vi "LS372_setup.vi"   [LabVIEW 2016]
uses:
  Instrument_Setup.vi
  Lake Shore 372/Lake Shore 372.lvlib
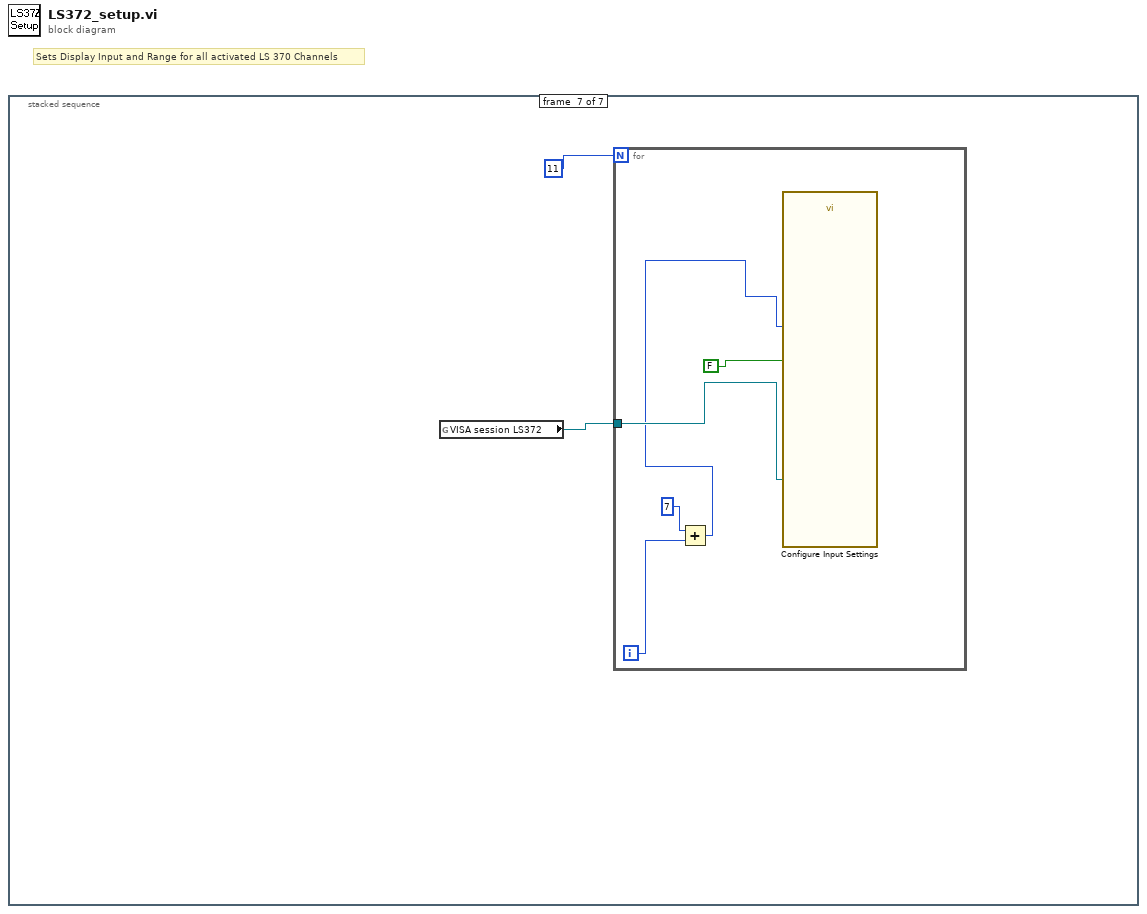
[diagram p0: block diagram]
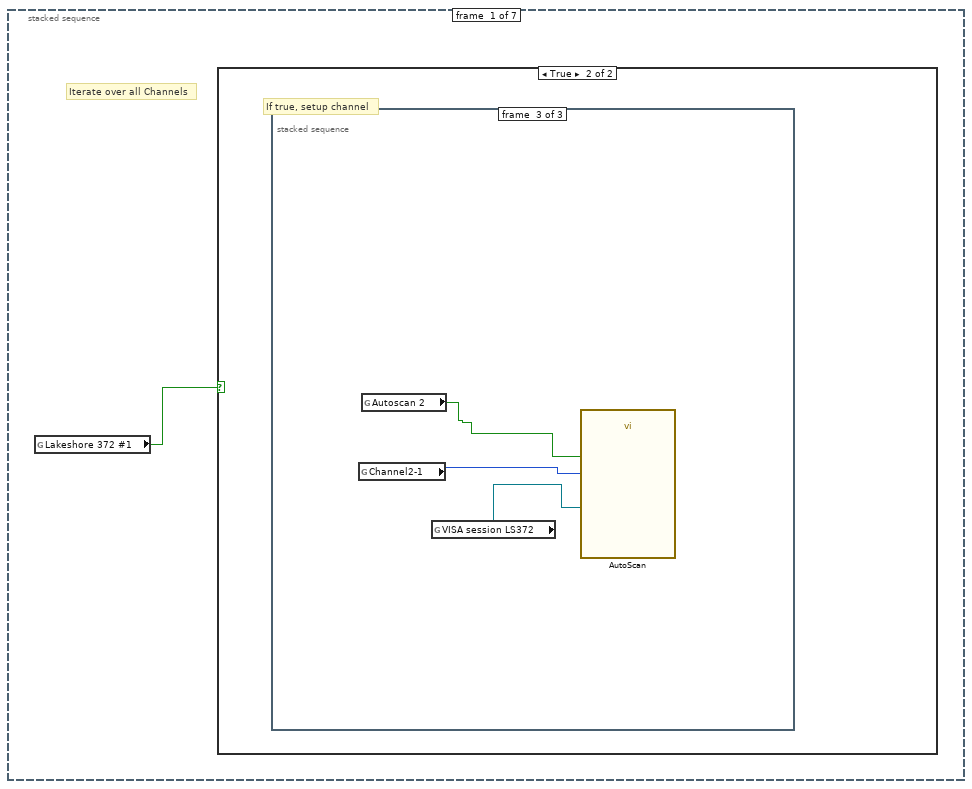
[diagram p2: hidden frame]
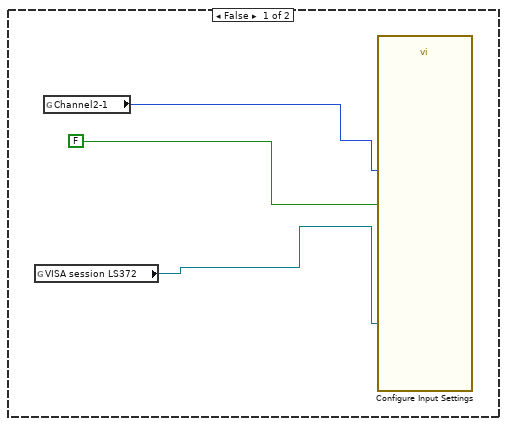
[diagram p3: hidden frame]
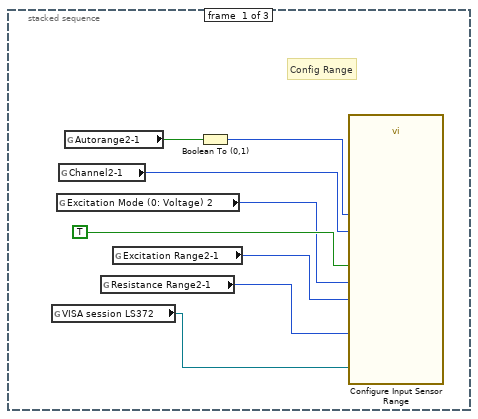
[diagram p4: hidden frame]
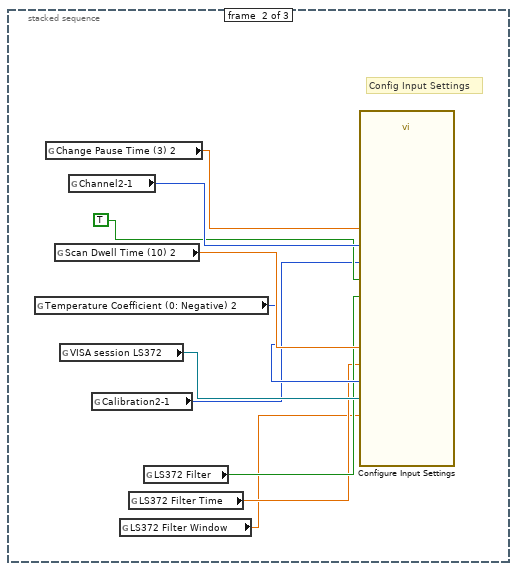
[diagram p5: hidden frame]
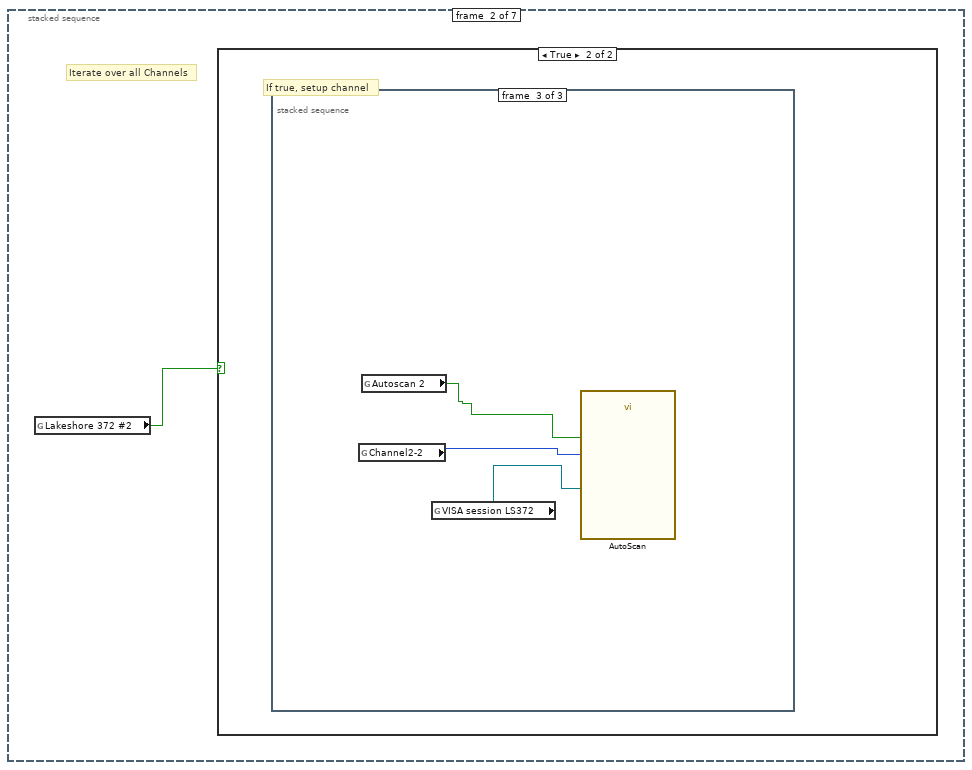
[diagram p6: hidden frame]
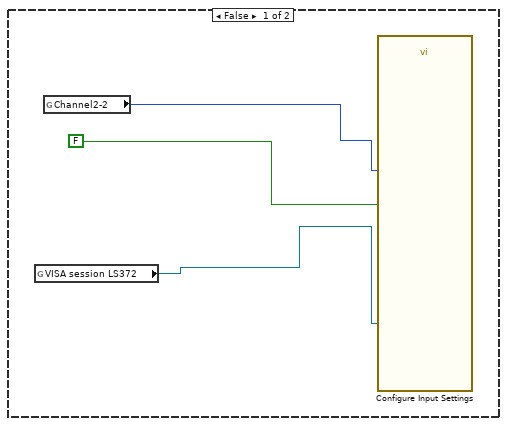
[diagram p7: hidden frame]
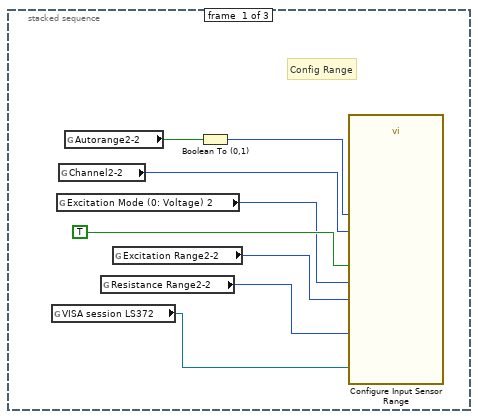
[diagram p8: hidden frame]
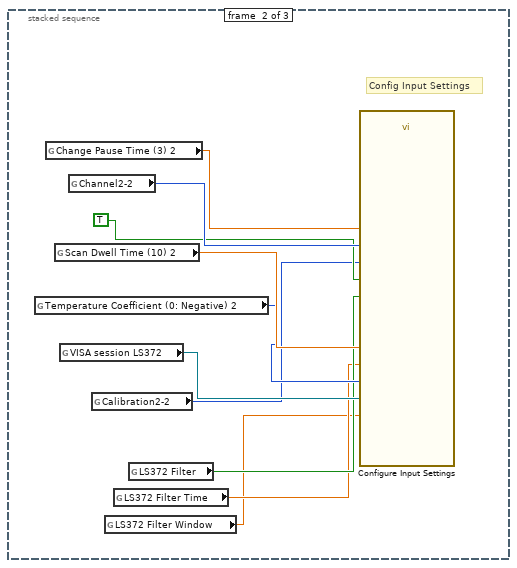
[diagram p9: hidden frame]
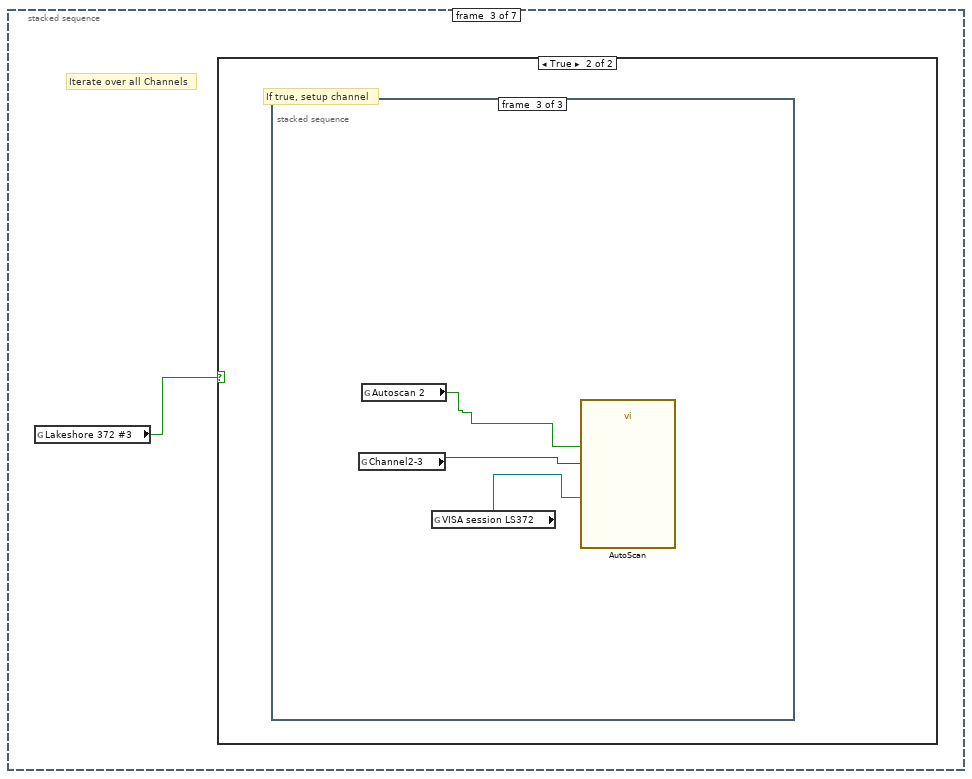
[diagram p10: hidden frame]
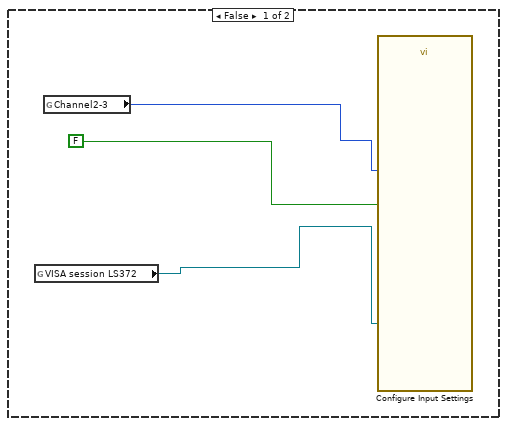
[diagram p11: hidden frame]
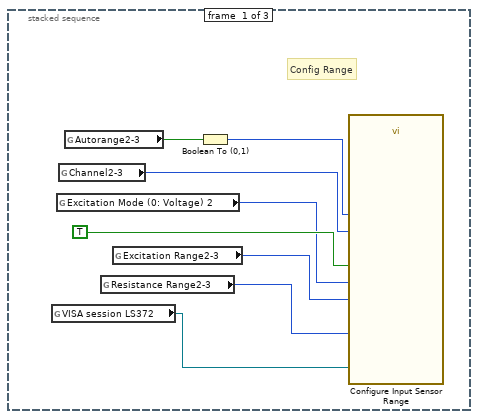
[diagram p12: hidden frame]
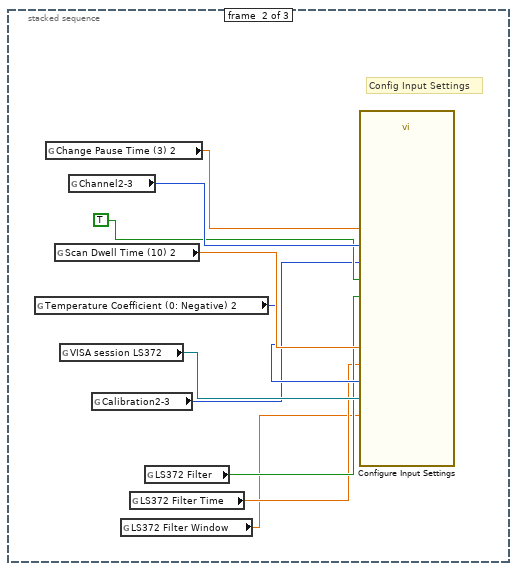
[diagram p13: hidden frame]
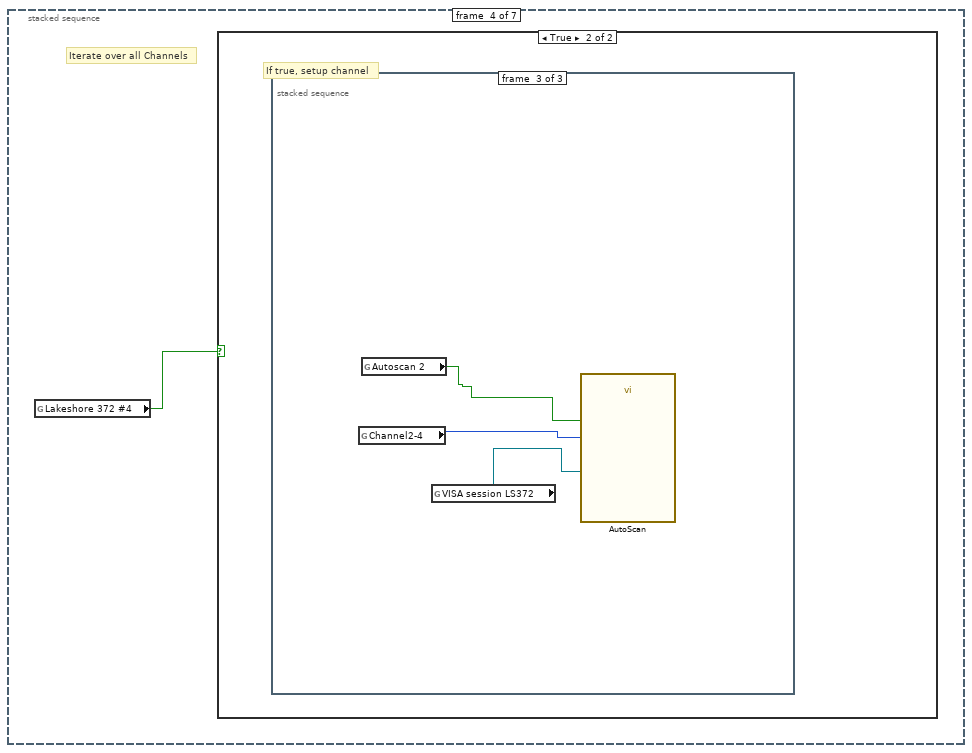
[diagram p14: hidden frame]
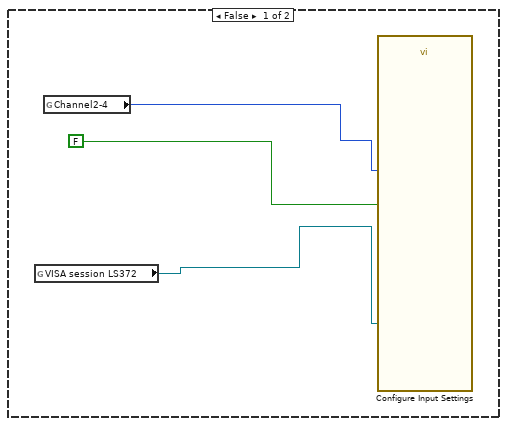
[diagram p15: hidden frame]
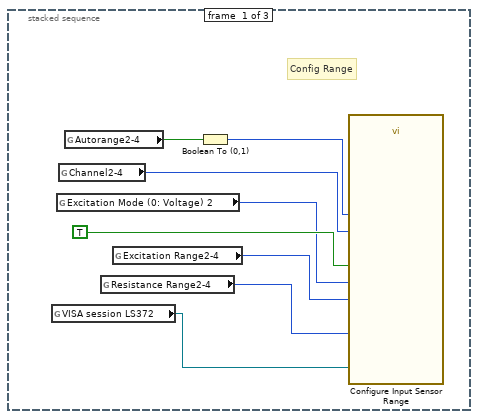
[diagram p16: hidden frame]
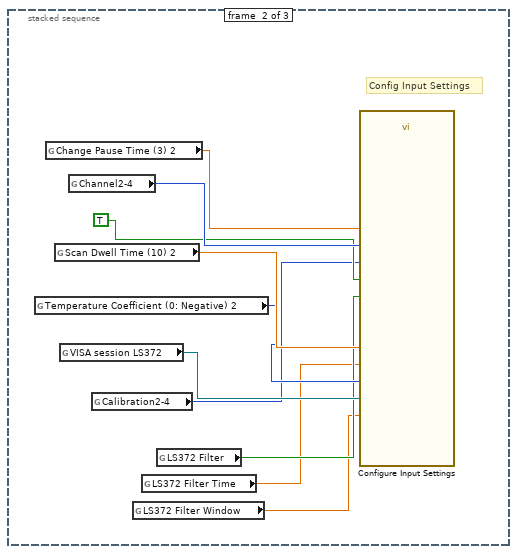
[diagram p17: hidden frame]
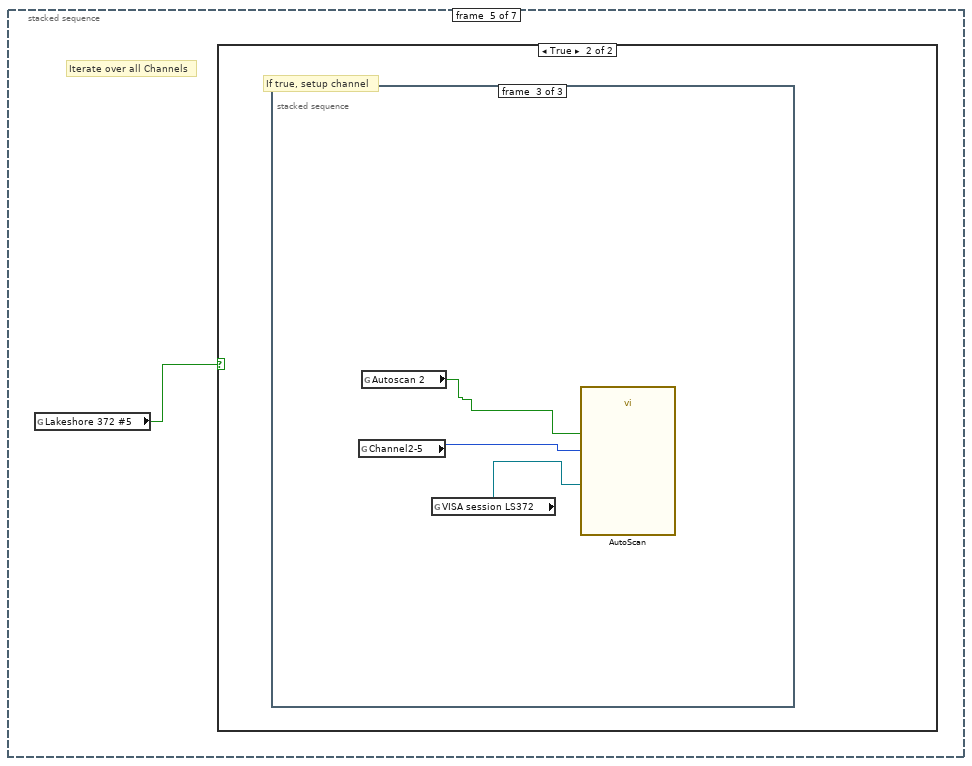
[diagram p18: hidden frame]
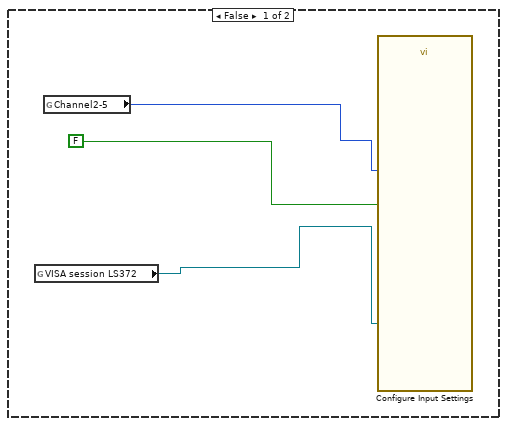
[diagram p19: hidden frame]
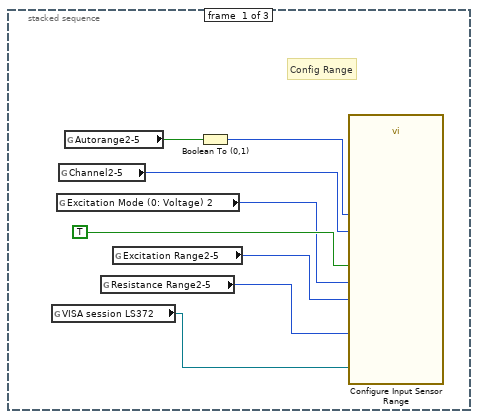
[diagram p20: hidden frame]
diagram:
  # "Sets Display Input and Range for all activated LS 370 Channels"
  n1 = stacked-sequence {
    frame #0 {
      # "Iterate over all Channels"
      n2 = global read "Instrument_Setup.vi" "Lakeshore 372 #1"() -> (w1:bool)
      n3 = case shown="True" w1 {
        frame False {
          n4 = global read "Instrument_Setup.vi" "VISA session LS372"() -> (w2:refnum<visa-resource-name>)
          n5 = global read "Instrument_Setup.vi" "Channel2-1"() -> (w4:u16)
          n6 = call "Configure Input Settings.vi"("VISA resource name"=w2, "Channel (1)"=w4, "Enable Channel (T: Enable)"=FALSE) -> ()  [unwired: 15 in, 2 out]
        }
        frame True {
          # "If true, setup channel"
          n7 = stacked-sequence {
            frame #0 {
              # "Config Range"
              n8 = global read "Instrument_Setup.vi" "VISA session LS372"() -> (w5:refnum<visa-resource-name>)
              n9 = global read "Instrument_Setup.vi" "Excitation Mode (0: Voltage) 2"() -> (w8:u16)
              n10 = global read "Instrument_Setup.vi" "Channel2-1"() -> (w10:u16)
              n11 = global read "Instrument_Setup.vi" "Autorange2-1"() -> (w12:bool)
              n12 = global read "Instrument_Setup.vi" "Resistance Range2-1"() -> (w6:u16)
              n13 = global read "Instrument_Setup.vi" "Excitation Range2-1"() -> (w7:u16)
              n14 = Boolean To (0,1)(Boolean=w12) -> (0, 1=w11:i16)
              n15 = call "Configure Input Sensor Range.vi"("VISA resource name"=w5, "Channel (1)"=w10, "Excitation Mode (0: Voltage)"=w8, "Excitation Range (5: 200 uV / 100 pA)"=w7, "Autorange (0: Autorange off)"=w11, "Resistance Range (17: 200 kOhm)"=w6, "Excitation  (T: On)"=TRUE) -> ()  [unwired: 11 in, 2 out]
            }
            frame #1 {
              # "Config Input Settings"
              n16 = global read "Instrument_Setup.vi" "Temperature Coefficient (0: Negative) 2"() -> (w18:u16)
              n17 = global read "Instrument_Setup.vi" "Change Pause Time (3) 2"() -> (w22:dbl)
              n18 = global read "Instrument_Setup.vi" "Scan Dwell Time (10) 2"() -> (w19:dbl)
              n19 = global read "Instrument_Setup.vi" "VISA session LS372"() -> (w17:refnum<visa-resource-name>)
              n20 = global read "Instrument_Setup.vi" "Channel2-1"() -> (w21:u16)
              n21 = global read "Instrument_Setup.vi" "Calibration2-1"() -> (w16:i32)
              n22 = global read "Instrument_Setup.vi" "LS372 Filter Window"() -> (w13:dbl)
              n23 = global read "Instrument_Setup.vi" "LS372 Filter Time"() -> (w14:dbl)
              n24 = global read "Instrument_Setup.vi" "LS372 Filter"() -> (w15:bool)
              n25 = call "Configure Input Settings.vi"("VISA resource name"=w17, "Channel (1)"=w21, "Scan Dwell Time (10)"=w19, "Change Pause Time (3)"=w22, "Curve Number (0)"=w16, "Enable Channel (T: Enable)"=TRUE, "Enable Filter (F: Off)"=w15, "Temperature Coefficient (1: Negative)"=w18, "Settle Time (10 sec)"=w14, "Window (40% FS)"=w13) -> ()  [unwired: 8 in, 2 out]
            }
            frame #2 {
              n26 = global read "Instrument_Setup.vi" "Channel2-1"() -> (w24:u16)
              n27 = global read "Instrument_Setup.vi" "Autoscan 2"() -> (w25:bool)
              n28 = global read "Instrument_Setup.vi" "VISA session LS372"() -> (w23:refnum<visa-resource-name>)
              n29 = call "AutoScan.vi"("Autoscan (F: Off)"=w25, "Channel (1:1)"=w24, "VISA resource name"=w23) -> ()  [unwired: 7 in, 2 out]
            }
          }
        }
      }
    }
    frame #1 {
      # "Iterate over all Channels"
      n30 = global read "Instrument_Setup.vi" "Lakeshore 372 #2"() -> (w26:bool)
      n31 = case shown="True" w26 {
        frame False {
          n32 = global read "Instrument_Setup.vi" "VISA session LS372"() -> (w27:refnum<visa-resource-name>)
          n33 = global read "Instrument_Setup.vi" "Channel2-2"() -> (w29:u16)
          n34 = call "Configure Input Settings.vi"("VISA resource name"=w27, "Channel (1)"=w29, "Enable Channel (T: Enable)"=FALSE) -> ()  [unwired: 15 in, 2 out]
        }
        frame True {
          # "If true, setup channel"
          n35 = stacked-sequence {
            frame #0 {
              # "Config Range"
              n36 = global read "Instrument_Setup.vi" "VISA session LS372"() -> (w30:refnum<visa-resource-name>)
              n37 = global read "Instrument_Setup.vi" "Excitation Mode (0: Voltage) 2"() -> (w33:u16)
              n38 = global read "Instrument_Setup.vi" "Channel2-2"() -> (w35:u16)
              n39 = global read "Instrument_Setup.vi" "Autorange2-2"() -> (w37:bool)
              n40 = global read "Instrument_Setup.vi" "Resistance Range2-2"() -> (w31:u16)
              n41 = global read "Instrument_Setup.vi" "Excitation Range2-2"() -> (w32:u16)
              n42 = Boolean To (0,1)(Boolean=w37) -> (0, 1=w36:i16)
              n43 = call "Configure Input Sensor Range.vi"("VISA resource name"=w30, "Channel (1)"=w35, "Excitation Mode (0: Voltage)"=w33, "Excitation Range (5: 200 uV / 100 pA)"=w32, "Autorange (0: Autorange off)"=w36, "Resistance Range (17: 200 kOhm)"=w31, "Excitation  (T: On)"=TRUE) -> ()  [unwired: 11 in, 2 out]
            }
            frame #1 {
              # "Config Input Settings"
              n44 = global read "Instrument_Setup.vi" "Temperature Coefficient (0: Negative) 2"() -> (w43:u16)
              n45 = global read "Instrument_Setup.vi" "Change Pause Time (3) 2"() -> (w47:dbl)
              n46 = global read "Instrument_Setup.vi" "Scan Dwell Time (10) 2"() -> (w44:dbl)
              n47 = global read "Instrument_Setup.vi" "VISA session LS372"() -> (w42:refnum<visa-resource-name>)
              n48 = global read "Instrument_Setup.vi" "Channel2-2"() -> (w46:u16)
              n49 = global read "Instrument_Setup.vi" "Calibration2-2"() -> (w41:i32)
              n50 = global read "Instrument_Setup.vi" "LS372 Filter Window"() -> (w38:dbl)
              n51 = global read "Instrument_Setup.vi" "LS372 Filter Time"() -> (w39:dbl)
              n52 = global read "Instrument_Setup.vi" "LS372 Filter"() -> (w40:bool)
              n53 = call "Configure Input Settings.vi"("VISA resource name"=w42, "Channel (1)"=w46, "Scan Dwell Time (10)"=w44, "Change Pause Time (3)"=w47, "Curve Number (0)"=w41, "Enable Channel (T: Enable)"=TRUE, "Enable Filter (F: Off)"=w40, "Temperature Coefficient (1: Negative)"=w43, "Settle Time (10 sec)"=w39, "Window (40% FS)"=w38) -> ()  [unwired: 8 in, 2 out]
            }
            frame #2 {
              n54 = global read "Instrument_Setup.vi" "Channel2-2"() -> (w49:u16)
              n55 = global read "Instrument_Setup.vi" "Autoscan 2"() -> (w50:bool)
              n56 = global read "Instrument_Setup.vi" "VISA session LS372"() -> (w48:refnum<visa-resource-name>)
              n57 = call "AutoScan.vi"("Autoscan (F: Off)"=w50, "Channel (1:1)"=w49, "VISA resource name"=w48) -> ()  [unwired: 7 in, 2 out]
            }
          }
        }
      }
    }
    frame #2 {
      # "Iterate over all Channels"
      n58 = global read "Instrument_Setup.vi" "Lakeshore 372 #3"() -> (w51:bool)
      n59 = case shown="True" w51 {
        frame False {
          n60 = global read "Instrument_Setup.vi" "VISA session LS372"() -> (w52:refnum<visa-resource-name>)
          n61 = global read "Instrument_Setup.vi" "Channel2-3"() -> (w54:u16)
          n62 = call "Configure Input Settings.vi"("VISA resource name"=w52, "Channel (1)"=w54, "Enable Channel (T: Enable)"=FALSE) -> ()  [unwired: 15 in, 2 out]
        }
        frame True {
          # "If true, setup channel"
          n63 = stacked-sequence {
            frame #0 {
              # "Config Range"
              n64 = global read "Instrument_Setup.vi" "VISA session LS372"() -> (w55:refnum<visa-resource-name>)
              n65 = global read "Instrument_Setup.vi" "Excitation Mode (0: Voltage) 2"() -> (w58:u16)
              n66 = global read "Instrument_Setup.vi" "Channel2-3"() -> (w60:u16)
              n67 = global read "Instrument_Setup.vi" "Autorange2-3"() -> (w62:bool)
              n68 = global read "Instrument_Setup.vi" "Resistance Range2-3"() -> (w56:u16)
              n69 = global read "Instrument_Setup.vi" "Excitation Range2-3"() -> (w57:u16)
              n70 = Boolean To (0,1)(Boolean=w62) -> (0, 1=w61:i16)
              n71 = call "Configure Input Sensor Range.vi"("VISA resource name"=w55, "Channel (1)"=w60, "Excitation Mode (0: Voltage)"=w58, "Excitation Range (5: 200 uV / 100 pA)"=w57, "Autorange (0: Autorange off)"=w61, "Resistance Range (17: 200 kOhm)"=w56, "Excitation  (T: On)"=TRUE) -> ()  [unwired: 11 in, 2 out]
            }
            frame #1 {
              # "Config Input Settings"
              n72 = global read "Instrument_Setup.vi" "Temperature Coefficient (0: Negative) 2"() -> (w68:u16)
              n73 = global read "Instrument_Setup.vi" "Change Pause Time (3) 2"() -> (w72:dbl)
              n74 = global read "Instrument_Setup.vi" "Scan Dwell Time (10) 2"() -> (w69:dbl)
              n75 = global read "Instrument_Setup.vi" "VISA session LS372"() -> (w67:refnum<visa-resource-name>)
              n76 = global read "Instrument_Setup.vi" "Channel2-3"() -> (w71:u16)
              n77 = global read "Instrument_Setup.vi" "Calibration2-3"() -> (w66:i32)
              n78 = global read "Instrument_Setup.vi" "LS372 Filter Window"() -> (w63:dbl)
              n79 = global read "Instrument_Setup.vi" "LS372 Filter Time"() -> (w64:dbl)
              n80 = global read "Instrument_Setup.vi" "LS372 Filter"() -> (w65:bool)
              n81 = call "Configure Input Settings.vi"("VISA resource name"=w67, "Channel (1)"=w71, "Scan Dwell Time (10)"=w69, "Change Pause Time (3)"=w72, "Curve Number (0)"=w66, "Enable Channel (T: Enable)"=TRUE, "Enable Filter (F: Off)"=w65, "Temperature Coefficient (1: Negative)"=w68, "Settle Time (10 sec)"=w64, "Window (40% FS)"=w63) -> ()  [unwired: 8 in, 2 out]
            }
            frame #2 {
              n82 = global read "Instrument_Setup.vi" "Channel2-3"() -> (w74:u16)
              n83 = global read "Instrument_Setup.vi" "Autoscan 2"() -> (w75:bool)
              n84 = global read "Instrument_Setup.vi" "VISA session LS372"() -> (w73:refnum<visa-resource-name>)
              n85 = call "AutoScan.vi"("Autoscan (F: Off)"=w75, "Channel (1:1)"=w74, "VISA resource name"=w73) -> ()  [unwired: 7 in, 2 out]
            }
          }
        }
      }
    }
    frame #3 {
      # "Iterate over all Channels"
      n86 = global read "Instrument_Setup.vi" "Lakeshore 372 #4"() -> (w76:bool)
      n87 = case shown="True" w76 {
        frame False {
          n88 = global read "Instrument_Setup.vi" "VISA session LS372"() -> (w77:refnum<visa-resource-name>)
          n89 = global read "Instrument_Setup.vi" "Channel2-4"() -> (w79:u16)
          n90 = call "Configure Input Settings.vi"("VISA resource name"=w77, "Channel (1)"=w79, "Enable Channel (T: Enable)"=FALSE) -> ()  [unwired: 15 in, 2 out]
        }
        frame True {
          # "If true, setup channel"
          n91 = stacked-sequence {
            frame #0 {
              # "Config Range"
              n92 = global read "Instrument_Setup.vi" "VISA session LS372"() -> (w80:refnum<visa-resource-name>)
              n93 = global read "Instrument_Setup.vi" "Excitation Mode (0: Voltage) 2"() -> (w83:u16)
              n94 = global read "Instrument_Setup.vi" "Channel2-4"() -> (w85:u16)
              n95 = global read "Instrument_Setup.vi" "Autorange2-4"() -> (w87:bool)
              n96 = global read "Instrument_Setup.vi" "Resistance Range2-4"() -> (w81:u16)
              n97 = global read "Instrument_Setup.vi" "Excitation Range2-4"() -> (w82:u16)
              n98 = Boolean To (0,1)(Boolean=w87) -> (0, 1=w86:i16)
              n99 = call "Configure Input Sensor Range.vi"("VISA resource name"=w80, "Channel (1)"=w85, "Excitation Mode (0: Voltage)"=w83, "Excitation Range (5: 200 uV / 100 pA)"=w82, "Autorange (0: Autorange off)"=w86, "Resistance Range (17: 200 kOhm)"=w81, "Excitation  (T: On)"=TRUE) -> ()  [unwired: 11 in, 2 out]
            }
            frame #1 {
              # "Config Input Settings"
              n100 = global read "Instrument_Setup.vi" "Temperature Coefficient (0: Negative) 2"() -> (w93:u16)
              n101 = global read "Instrument_Setup.vi" "Change Pause Time (3) 2"() -> (w97:dbl)
              n102 = global read "Instrument_Setup.vi" "Scan Dwell Time (10) 2"() -> (w94:dbl)
              n103 = global read "Instrument_Setup.vi" "VISA session LS372"() -> (w92:refnum<visa-resource-name>)
              n104 = global read "Instrument_Setup.vi" "Channel2-4"() -> (w96:u16)
              n105 = global read "Instrument_Setup.vi" "Calibration2-4"() -> (w91:i32)
              n106 = global read "Instrument_Setup.vi" "LS372 Filter Window"() -> (w88:dbl)
              n107 = global read "Instrument_Setup.vi" "LS372 Filter Time"() -> (w89:dbl)
              n108 = global read "Instrument_Setup.vi" "LS372 Filter"() -> (w90:bool)
              n109 = call "Configure Input Settings.vi"("VISA resource name"=w92, "Channel (1)"=w96, "Scan Dwell Time (10)"=w94, "Change Pause Time (3)"=w97, "Curve Number (0)"=w91, "Enable Channel (T: Enable)"=TRUE, "Enable Filter (F: Off)"=w90, "Temperature Coefficient (1: Negative)"=w93, "Settle Time (10 sec)"=w89, "Window (40% FS)"=w88) -> ()  [unwired: 8 in, 2 out]
            }
            frame #2 {
              n110 = global read "Instrument_Setup.vi" "Channel2-4"() -> (w99:u16)
              n111 = global read "Instrument_Setup.vi" "Autoscan 2"() -> (w100:bool)
              n112 = global read "Instrument_Setup.vi" "VISA session LS372"() -> (w98:refnum<visa-resource-name>)
              n113 = call "AutoScan.vi"("Autoscan (F: Off)"=w100, "Channel (1:1)"=w99, "VISA resource name"=w98) -> ()  [unwired: 7 in, 2 out]
            }
          }
        }
      }
    }
    frame #4 {
      # "Iterate over all Channels"
      n114 = global read "Instrument_Setup.vi" "Lakeshore 372 #5"() -> (w101:bool)
      n115 = case shown="True" w101 {
        frame False {
          n116 = global read "Instrument_Setup.vi" "VISA session LS372"() -> (w102:refnum<visa-resource-name>)
          n117 = global read "Instrument_Setup.vi" "Channel2-5"() -> (w104:u16)
          n118 = call "Configure Input Settings.vi"("VISA resource name"=w102, "Channel (1)"=w104, "Enable Channel (T: Enable)"=FALSE) -> ()  [unwired: 15 in, 2 out]
        }
        frame True {
          # "If true, setup channel"
          n119 = stacked-sequence {
            frame #0 {
              # "Config Range"
              n120 = global read "Instrument_Setup.vi" "VISA session LS372"() -> (w105:refnum<visa-resource-name>)
              n121 = global read "Instrument_Setup.vi" "Excitation Mode (0: Voltage) 2"() -> (w108:u16)
              n122 = global read "Instrument_Setup.vi" "Channel2-5"() -> (w110:u16)
              n123 = global read "Instrument_Setup.vi" "Autorange2-5"() -> (w112:bool)
              n124 = global read "Instrument_Setup.vi" "Resistance Range2-5"() -> (w106:u16)
              n125 = global read "Instrument_Setup.vi" "Excitation Range2-5"() -> (w107:u16)
              n126 = Boolean To (0,1)(Boolean=w112) -> (0, 1=w111:i16)
              n127 = call "Configure Input Sensor Range.vi"("VISA resource name"=w105, "Channel (1)"=w110, "Excitation Mode (0: Voltage)"=w108, "Excitation Range (5: 200 uV / 100 pA)"=w107, "Autorange (0: Autorange off)"=w111, "Resistance Range (17: 200 kOhm)"=w106, "Excitation  (T: On)"=TRUE) -> ()  [unwired: 11 in, 2 out]
            }
            frame #1 {
              # "Config Input Settings"
              n128 = global read "Instrument_Setup.vi" "Temperature Coefficient (0: Negative) 2"() -> (w118:u16)
              n129 = global read "Instrument_Setup.vi" "Change Pause Time (3) 2"() -> (w122:dbl)
              n130 = global read "Instrument_Setup.vi" "Scan Dwell Time (10) 2"() -> (w119:dbl)
              n131 = global read "Instrument_Setup.vi" "VISA session LS372"() -> (w117:refnum<visa-resource-name>)
              n132 = global read "Instrument_Setup.vi" "Channel2-5"() -> (w121:u16)
              n133 = global read "Instrument_Setup.vi" "LS372 Filter Window"() -> (w113:dbl)
              n134 = global read "Instrument_Setup.vi" "LS372 Filter Time"() -> (w114:dbl)
              n135 = global read "Instrument_Setup.vi" "Calibration2-5"() -> (w116:i32)
              n136 = global read "Instrument_Setup.vi" "LS372 Filter"() -> (w115:bool)
              n137 = call "Configure Input Settings.vi"("VISA resource name"=w117, "Channel (1)"=w121, "Scan Dwell Time (10)"=w119, "Change Pause Time (3)"=w122, "Curve Number (0)"=w116, "Enable Channel (T: Enable)"=TRUE, "Enable Filter (F: Off)"=w115, "Temperature Coefficient (1: Negative)"=w118, "Settle Time (10 sec)"=w114, "Window (40% FS)"=w113) -> ()  [unwired: 8 in, 2 out]
            }
            frame #2 {
              n138 = global read "Instrument_Setup.vi" "Channel2-5"() -> (w124:u16)
              n139 = global read "Instrument_Setup.vi" "Autoscan 2"() -> (w125:bool)
              n140 = global read "Instrument_Setup.vi" "VISA session LS372"() -> (w123:refnum<visa-resource-name>)
              n141 = call "AutoScan.vi"("Autoscan (F: Off)"=w125, "Channel (1:1)"=w124, "VISA resource name"=w123) -> ()  [unwired: 7 in, 2 out]
            }
          }
        }
      }
    }
    frame #5 {
      # "Iterate over all Channels"
      n142 = global read "Instrument_Setup.vi" "Lakeshore 372 #6"() -> (w126:bool)
      n143 = case shown="True" w126 {
        frame False {
          n144 = global read "Instrument_Setup.vi" "VISA session LS372"() -> (w127:refnum<visa-resource-name>)
          n145 = global read "Instrument_Setup.vi" "Channel2-6"() -> (w129:u16)
          n146 = call "Configure Input Settings.vi"("VISA resource name"=w127, "Channel (1)"=w129, "Enable Channel (T: Enable)"=FALSE) -> ()  [unwired: 15 in, 2 out]
        }
        frame True {
          # "If true, setup channel"
          n147 = stacked-sequence {
            frame #0 {
              # "Config Range"
              n148 = global read "Instrument_Setup.vi" "VISA session LS372"() -> (w130:refnum<visa-resource-name>)
              n149 = global read "Instrument_Setup.vi" "Excitation Mode (0: Voltage) 2"() -> (w133:u16)
              n150 = global read "Instrument_Setup.vi" "Channel2-6"() -> (w135:u16)
              n151 = global read "Instrument_Setup.vi" "Autorange2-6"() -> (w137:bool)
              n152 = global read "Instrument_Setup.vi" "Resistance Range2-6"() -> (w131:u16)
              n153 = global read "Instrument_Setup.vi" "Excitation Range2-6"() -> (w132:u16)
              n154 = Boolean To (0,1)(Boolean=w137) -> (0, 1=w136:i16)
              n155 = call "Configure Input Sensor Range.vi"("VISA resource name"=w130, "Channel (1)"=w135, "Excitation Mode (0: Voltage)"=w133, "Excitation Range (5: 200 uV / 100 pA)"=w132, "Autorange (0: Autorange off)"=w136, "Resistance Range (17: 200 kOhm)"=w131, "Excitation  (T: On)"=TRUE) -> ()  [unwired: 11 in, 2 out]
            }
            frame #1 {
              # "Config Input Settings"
              n156 = global read "Instrument_Setup.vi" "Temperature Coefficient (0: Negative) 2"() -> (w143:u16)
              n157 = global read "Instrument_Setup.vi" "Change Pause Time (3) 2"() -> (w147:dbl)
              n158 = global read "Instrument_Setup.vi" "Scan Dwell Time (10) 2"() -> (w144:dbl)
              n159 = global read "Instrument_Setup.vi" "VISA session LS372"() -> (w142:refnum<visa-resource-name>)
              n160 = global read "Instrument_Setup.vi" "Channel2-6"() -> (w146:u16)
              n161 = global read "Instrument_Setup.vi" "Calibration2-6"() -> (w141:i32)
              n162 = global read "Instrument_Setup.vi" "LS372 Filter Window"() -> (w138:dbl)
              n163 = global read "Instrument_Setup.vi" "LS372 Filter Time"() -> (w139:dbl)
              n164 = global read "Instrument_Setup.vi" "LS372 Filter"() -> (w140:bool)
              n165 = call "Configure Input Settings.vi"("VISA resource name"=w142, "Channel (1)"=w146, "Scan Dwell Time (10)"=w144, "Change Pause Time (3)"=w147, "Curve Number (0)"=w141, "Enable Channel (T: Enable)"=TRUE, "Enable Filter (F: Off)"=w140, "Temperature Coefficient (1: Negative)"=w143, "Settle Time (10 sec)"=w139, "Window (40% FS)"=w138) -> ()  [unwired: 8 in, 2 out]
            }
            frame #2 {
              n166 = global read "Instrument_Setup.vi" "Channel2-6"() -> (w149:u16)
              n167 = global read "Instrument_Setup.vi" "Autoscan 2"() -> (w150:bool)
              n168 = global read "Instrument_Setup.vi" "VISA session LS372"() -> (w148:refnum<visa-resource-name>)
              n169 = call "AutoScan.vi"("Autoscan (F: Off)"=w150, "Channel (1:1)"=w149, "VISA resource name"=w148) -> ()  [unwired: 7 in, 2 out]
            }
          }
        }
      }
    }
    frame #6 {
      n170 = global read "Instrument_Setup.vi" "VISA session LS372"() -> (w152:refnum<visa-resource-name>)
      n171 = for {
        N: 11 -> [_]
        tunnel: w152 -> [w157]
        i -> [w154]
        n172 = Add(x=7, y=w154) -> (x+y=w153:i32)
        n173 = call "Configure Input Settings.vi"("VISA resource name"=w157, "Channel (1)"=w153, "Enable Channel (T: Enable)"=FALSE) -> ()  [unwired: 15 in, 2 out]
      }
    }
  }
